vi "DblToGStringArray.vi"(1 "Array":dbl[](array[numeric])) -> (0 "Array 2":string[](array[string]))   [LabVIEW 2024]
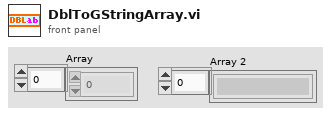
[diagram p1: front panel]
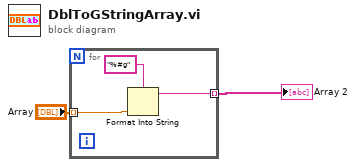
[diagram p0: block diagram]
diagram:
  n1 = for {
    tunnel: "Array" -> [w4] mode=indexing
    tunnel: [w3] -> w1 mode=indexing
    n2 = Format Into String(format string="%#g", w4) -> (resulting string=w3:string)  [unwired: 2 in, 1 out]
  }
  "Array 2" <- w1
